vi "Logarithm Data.vi"(8 "error in (no error)":errorcluster, 9 "Multiplot Representation In":T2, 10 "Actual Transform In":T6, 11 "3D Plot.lvclass in":refnum<class "3D Plot.lvclass">) -> (0 "error out":errorcluster, 1 "Multiplot Representation In":T2, 2 "Actual Transform Out":T6, 3 "3D Plot.lvclass out":refnum<class "3D Plot.lvclass">, 4 "Range Cluster":T1)   [LabVIEW 2017, in "3D Plot.lvclass"]
uses:
  <vilib>/Math Plots/3D Math Plots/3D Plot/3D Plot/3D Plot.lvclass
  <vilib>/Math Plots/3D Math Plots/3D Plot/3D Plot/Typedef/Actual Transform.ctl
  <vilib>/Math Plots/3D Math Plots/3D Plot/3D Plot/Typedef/Range Clusters.ctl
  <vilib>/Math Plots/3D Math Plots/3D Plot/3D Plot/Typedef/Multiplot Representation.ctl
  <vilib>/Math Plots/3D Math Plots/3D Plot/3D Plot/Typedef/Plot Representation.ctl
  <vilib>/Math Plots/3D Math Plots/3D Plot/3D Plot/Typedef/Mesh Data.ctl
  <vilib>/Math Plots/3D Math Plots/3D Plot/3D Plot/3D Plot.lvclass/3D Plot.ctl
  <vilib>/Math Plots/3D Math Plots/3D Plot/3D Plot Datatype/3D Plot Datatype.lvclass
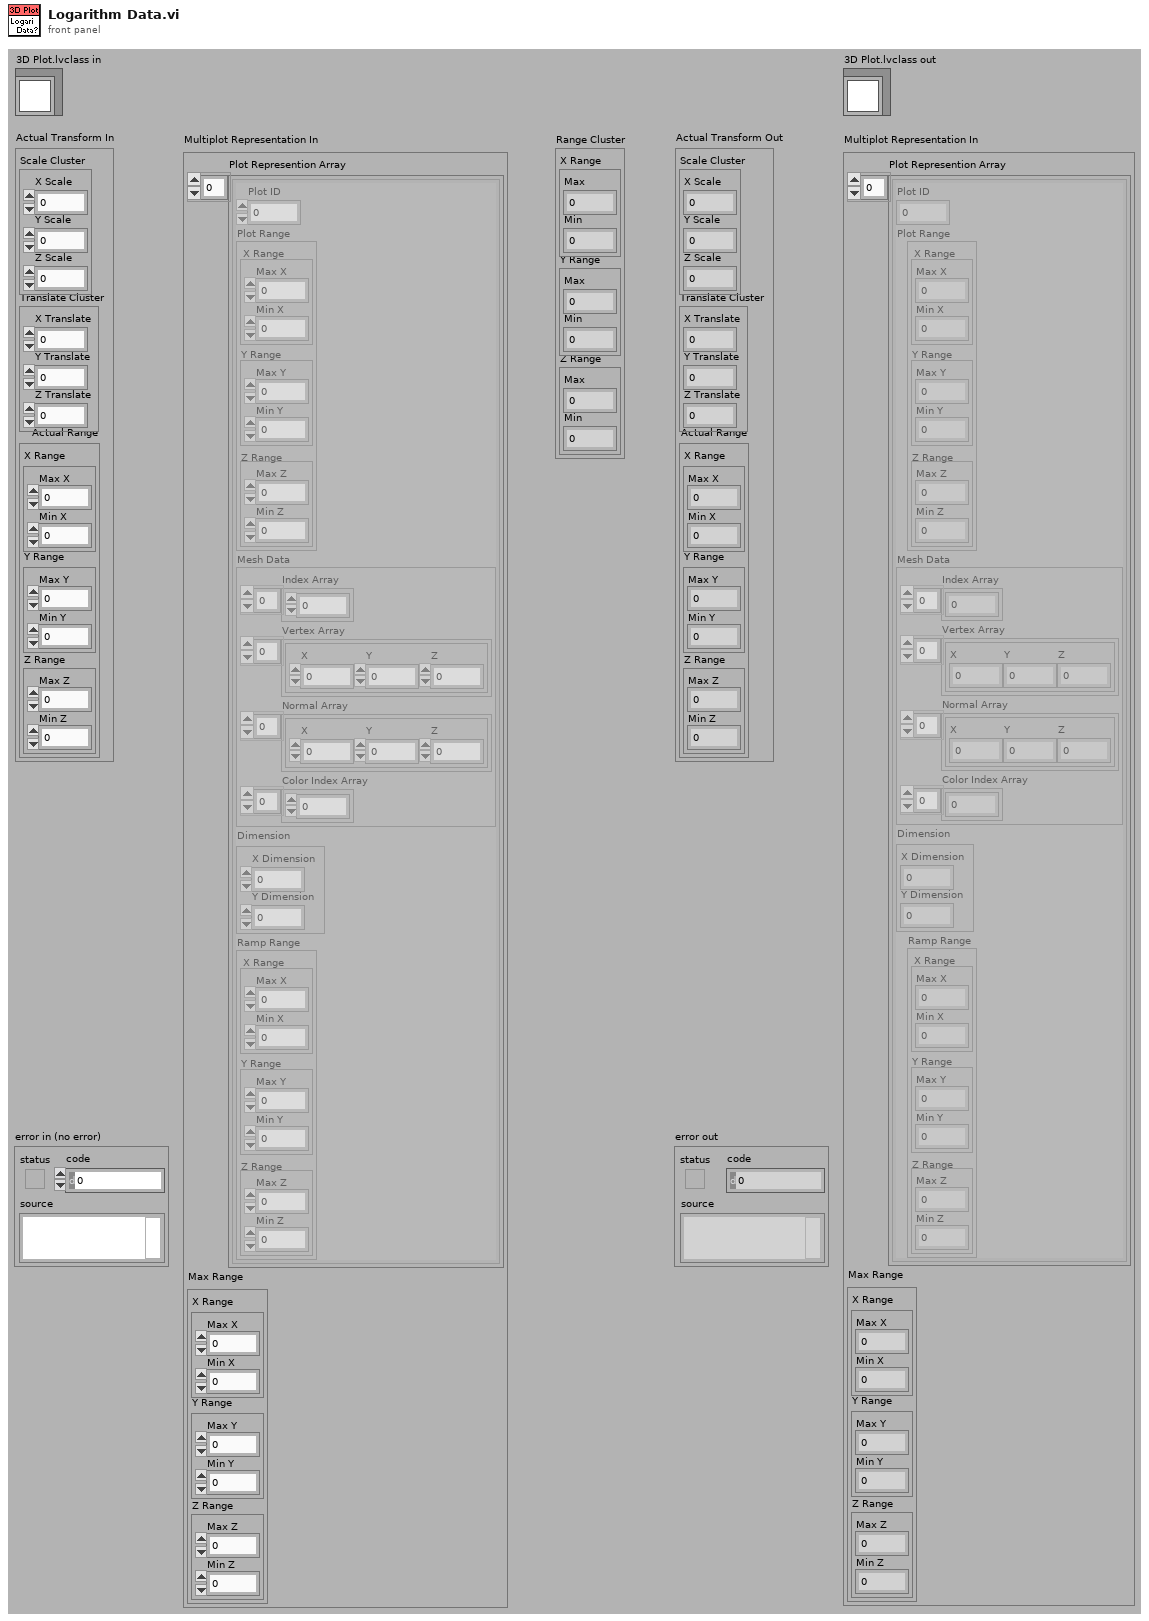
[diagram p1: front panel]
types:
  T1 = cluster{"X Range":cluster{"Max":sgl, "Min":sgl}, "Y Range":cluster{"Max":sgl, "Min":sgl}, "Z Range":cluster{"Max":sgl, "Min":sgl}}
  T2 = typedef "3D Plot.lvclass/Multiplot Representation.ctl" = cluster{"Plot Represention Array":T3[], "Max Range":T4}
  T3 = typedef "3D Plot.lvclass/Plot Representation.ctl" = cluster{"Plot ID":i32, "Plot Range":T4, "Mesh Data":T5, "Dimension":cluster{"X Dimension":i32, "Y Dimension":i32}, "Ramp Range":T4}
  T4 = typedef "3D Plot.lvclass/Range Clusters.ctl" = cluster{"X Range":cluster{"Max X":sgl, "Min X":sgl}, "Y Range":cluster{"Max Y":sgl, "Min Y":sgl}, "Z Range":cluster{"Max Z":sgl, "Min Z":sgl}}
  T5 = typedef "3D Plot.lvclass/Mesh Data.ctl" = cluster{"Index Array":u32[], "Vertex Array":cluster{"X":sgl, "Y":sgl, "Z":sgl}[], "Normal Array":cluster{"X":sgl, "Y":sgl, "Z":sgl}[], "Color Index Array":i32[]}
  T6 = typedef "3D Plot.lvclass/Actual Transform.ctl" = cluster{"Scale Cluster":cluster{"X Scale":sgl, "Y Scale":sgl, "Z Scale":sgl}, "Translate Cluster":cluster{"X Translate":sgl, "Y Translate":sgl, "Z Translate":sgl}, "Actual Range":T4}
  T7 = cluster{"Logarithm X":bool, "Logarithm Y":bool, "Logarithm Z":bool}
  T8 = cluster{"Range Out":cluster{"Max":sgl, "Min":sgl}, "Range Out":cluster{"Max":sgl, "Min":sgl}, "Range Out":cluster{"Max":sgl, "Min":sgl}}
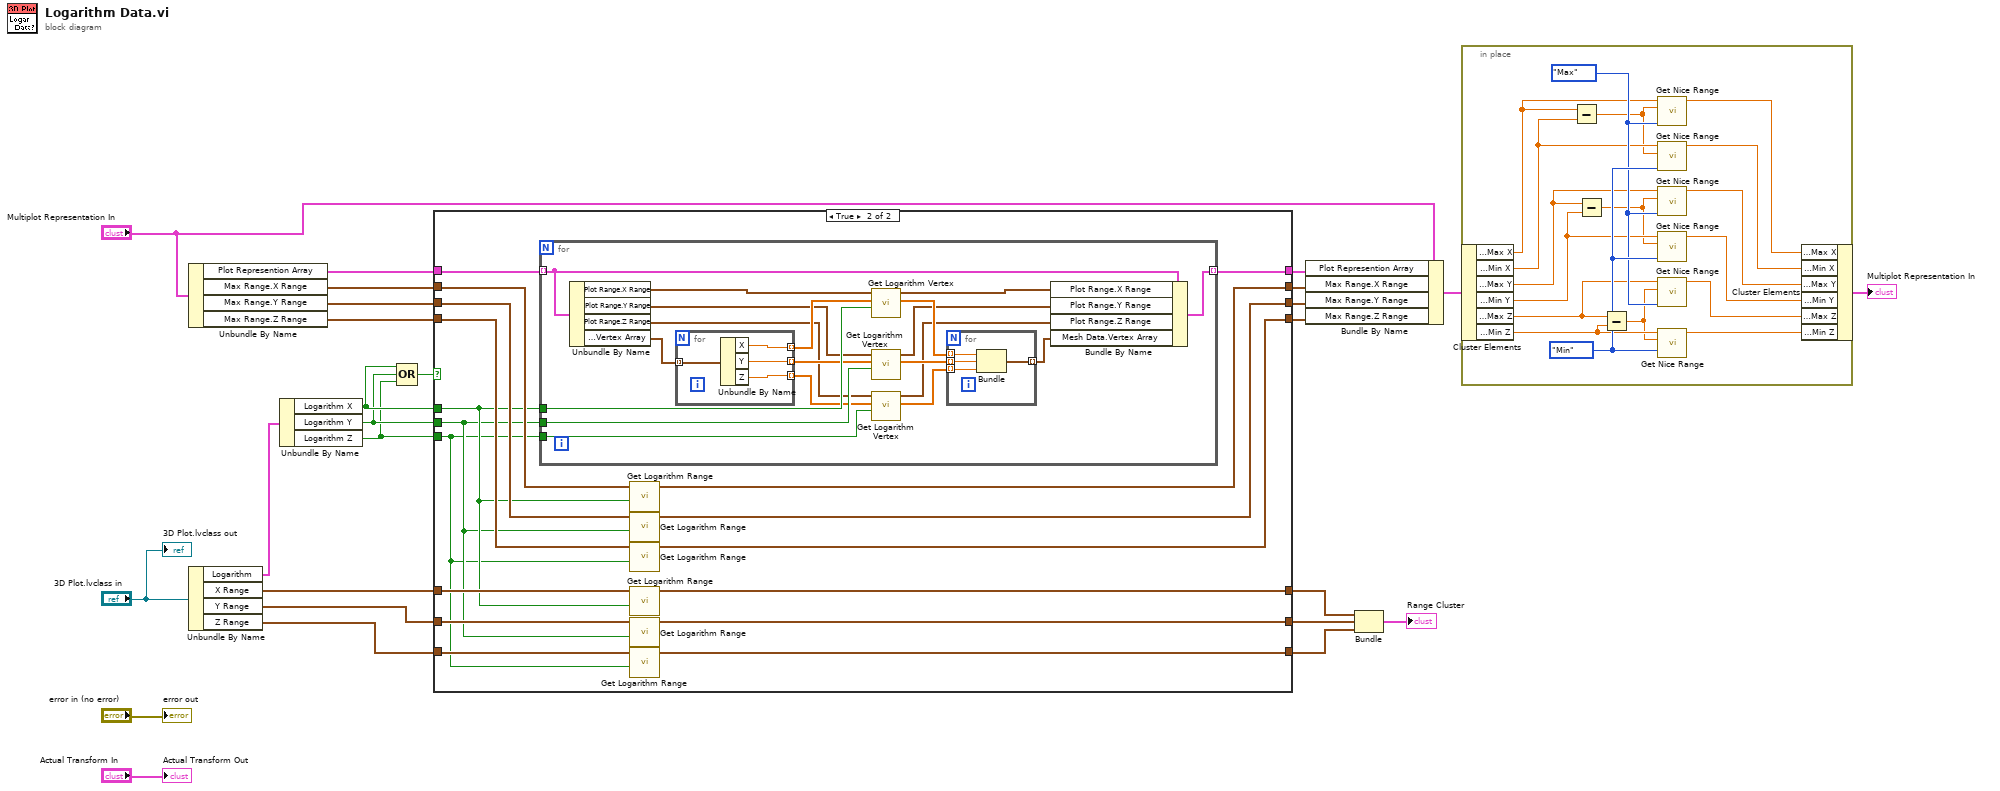
[diagram p0: block diagram]
diagram:
  n1 = Unbundle By Name("Multiplot Representation In") -> ("Plot Represention Array"=w17:T3[], "Max Range.X Range"=w15:cluster{"Max X":sgl, "Min X":sgl}, "Max Range.Y Range"=w14:cluster{"Max Y":sgl, "Min Y":sgl}, "Max Range.Z Range"=w13:cluster{"Max Z":sgl, "Min Z":sgl})
  n2 = Unbundle By Name("3D Plot.lvclass in") -> ("Logarithm"=w6:T7, "X Range"=w12:cluster{"Max X":sgl, "Min X":sgl}, "Y Range"=w11:cluster{"Max Y":sgl, "Min Y":sgl}, "Z Range"=w10:cluster{"Max Z":sgl, "Min Z":sgl})
  n3 = Unbundle By Name(w6) -> ("Logarithm X"=w21:bool, "Logarithm Y"=w20:bool, "Logarithm Z"=w19:bool)
  n4 = Compound Arithmetic op=OR(w21, w20, w19) -> (w18:bool)
  n5 = case shown="True" w18 {
    tunnel: w17 -> [w33 w50]
    tunnel: [w33 w49] -> w16
    tunnel: w21 -> [_ w36]
    tunnel: w20 -> [_ w35]
    tunnel: w19 -> [_ w34]
    tunnel: w15 -> [w32 w43]
    tunnel: w14 -> [w31 w47]
    tunnel: w13 -> [w30 w44]
    tunnel: w12 -> [w29 w42]
    tunnel: w11 -> [w28 w41]
    tunnel: w10 -> [w27 w40]
    tunnel: [w32 w48] -> w9
    tunnel: [w31 w46] -> w8
    tunnel: [w30 w45] -> w7
    tunnel: [w29 w37] -> w5
    tunnel: [w28 w38] -> w4
    tunnel: [w27 w39] -> w3
    frame False {
    }
    frame True {
      n6 = for {
        tunnel: w50 -> [w68] mode=indexing
        tunnel: [w69] -> w49 mode=indexing
        tunnel: w36 -> [w61]
        tunnel: w35 -> [w59]
        tunnel: w34 -> [w51]
        n7 = Unbundle By Name(w68) -> ("Plot Range.X Range"=w62:cluster{"Max X":sgl, "Min X":sgl}, "Plot Range.Y Range"=w60:cluster{"Max Y":sgl, "Min Y":sgl}, "Plot Range.Z Range"=w55:cluster{"Max Z":sgl, "Min Z":sgl}, "Mesh Data.Vertex Array"=w67:cluster{"X":sgl, "Y":sgl, "Z":sgl}[])
        n8 = for {
          tunnel: w67 -> [w77] mode=indexing
          tunnel: [w76] -> w66 mode=indexing
          tunnel: [w75] -> w58 mode=indexing
          tunnel: [w74] -> w54 mode=indexing
          n9 = Unbundle By Name(w77) -> ("X"=w76:sgl, "Y"=w75:sgl, "Z"=w74:sgl)
        }
        n10 = call <vilib>:"Get Logarithm Vertex.vi"("Logarithm?"=w61, "Vertex Array In"=w66, "Range In"=w62) -> ("Vertex Array Out"=w65:sgl[], "Range Out"=w63:cluster{"Max":sgl, "Min":sgl})  [unwired: 7 out]
        n11 = call <vilib>:"Get Logarithm Vertex.vi"("Logarithm?"=w59, "Vertex Array In"=w58, "Range In"=w60) -> ("Vertex Array Out"=w56:sgl[], "Range Out"=w57:cluster{"Max":sgl, "Min":sgl})  [unwired: 7 out]
        n12 = call <vilib>:"Get Logarithm Vertex.vi"("Logarithm?"=w51, "Vertex Array In"=w54, "Range In"=w55) -> ("Vertex Array Out"=w52:sgl[], "Range Out"=w53:cluster{"Max":sgl, "Min":sgl})  [unwired: 7 out]
        n13 = for {
          tunnel: [w73] -> w64 mode=indexing
          tunnel: w65 -> [w72] mode=indexing
          tunnel: w52 -> [w71] mode=indexing
          tunnel: w56 -> [w70] mode=indexing
          n14 = Bundle("X"=w72, "X"=w70, "X"=w71) -> (w73:cluster{"X":sgl, "X":sgl, "X":sgl})  [unwired: 1 out]
        }
        n15 = Bundle By Name(cluster=w68, "Plot Range.X Range"=w63, "Plot Range.Y Range"=w57, "Plot Range.Z Range"=w53, "Mesh Data.Vertex Array"=w64) -> (w69:T3)
      }
      n16 = call <vilib>:"Get Logarithm Range.vi"("Logarithm?"=w36, "Range In"=w43) -> ("Range Out"=w48:cluster{"Max":sgl, "Min":sgl})  [unwired: 3 in, 6 out]
      n17 = call <vilib>:"Get Logarithm Range.vi"("Logarithm?"=w35, "Range In"=w47) -> ("Range Out"=w46:cluster{"Max":sgl, "Min":sgl})  [unwired: 3 in, 6 out]
      n18 = call <vilib>:"Get Logarithm Range.vi"("Logarithm?"=w34, "Range In"=w44) -> ("Range Out"=w45:cluster{"Max":sgl, "Min":sgl})  [unwired: 2 in, 7 out]
      n19 = call <vilib>:"Get Logarithm Range.vi"("Logarithm?"=w36, "Range In"=w42) -> ("Range Out"=w37:cluster{"Max":sgl, "Min":sgl})  [unwired: 2 in, 7 out]
      n20 = call <vilib>:"Get Logarithm Range.vi"("Logarithm?"=w35, "Range In"=w41) -> ("Range Out"=w38:cluster{"Max":sgl, "Min":sgl})  [unwired: 2 in, 7 out]
      n21 = call <vilib>:"Get Logarithm Range.vi"("Logarithm?"=w34, "Range In"=w40) -> ("Range Out"=w39:cluster{"Max":sgl, "Min":sgl})  [unwired: 2 in, 7 out]
    }
  }
  n22 = Bundle By Name(cluster="Multiplot Representation In", "Plot Represention Array"=w16, "Max Range.X Range"=w9, "Max Range.Y Range"=w8, "Max Range.Z Range"=w7) -> (w2:T2)
  n23 = Bundle("Range Out"=w5, "Range Out"=w4, "Range Out"=w3) -> (→"Range Cluster":T8)  [unwired: 1 out]
  n24 = in-place {
    w87 = enum16{"Max", "Min"}."Max" ("Type")
    w88 = enum16{"Max", "Min"}."Min" ("Type")
    n25 = in-place-cluster #1(w2) -> ("Max Range.X Range.Max X"=w86:sgl, "Max Range.X Range.Min X"=w85:sgl, "Max Range.Y Range.Max Y"=w84:sgl, "Max Range.Y Range.Min Y"=w83:sgl, "Max Range.Z Range.Max Z"=w82:sgl, "Max Range.Z Range.Min Z"=w81:sgl)
    n26 = Subtract(x=w86, y=w85) -> (x-y=w80:sgl)
    n27 = Subtract(x=w84, y=w83) -> (x-y=w79:sgl)
    n28 = Subtract(x=w82, y=w81) -> (x-y=w78:sgl)
    n29 = call <vilib>:"Get Nice Range.vi"("Type"=w87, "Difference"=w80, "Input"=w86) -> ("Output"=w94:sgl)  [unwired: 8 out]
    n30 = call <vilib>:"Get Nice Range.vi"("Type"=w88, "Difference"=w80, "Input"=w85) -> ("Output"=w93:sgl)  [unwired: 8 out]
    n31 = call <vilib>:"Get Nice Range.vi"("Type"=w87, "Difference"=w79, "Input"=w84) -> ("Output"=w92:sgl)  [unwired: 8 out]
    n32 = call <vilib>:"Get Nice Range.vi"("Type"=w88, "Difference"=w79, "Input"=w83) -> ("Output"=w91:sgl)  [unwired: 8 out]
    n33 = call <vilib>:"Get Nice Range.vi"("Type"=w87, "Difference"=w78, "Input"=w82) -> ("Output"=w90:sgl)  [unwired: 8 out]
    n34 = call <vilib>:"Get Nice Range.vi"("Type"=w88, "Difference"=w78, "Input"=w81) -> ("Output"=w89:sgl)  [unwired: 8 out]
    n35 = in-place-cluster #1("Max Range.X Range.Max X"=w94, "Max Range.X Range.Min X"=w93, "Max Range.Y Range.Max Y"=w92, "Max Range.Y Range.Min Y"=w91, "Max Range.Z Range.Max Z"=w90, "Max Range.Z Range.Min Z"=w89) -> (→"Multiplot Representation In":T2)
  }
  "error out" <- "error in (no error)"
  "Actual Transform Out" <- "Actual Transform In"
  "3D Plot.lvclass out" <- "3D Plot.lvclass in"
